vi "Assess Message Type.vi"(10 "Command Word":u16 format="%04x", 11 "Status Word":u16 format="%04x") -> (3 "Message Type":T1)   [LabVIEW 2016, in "BCI-1553 API.lvlib" / "Bus Monitor.lvclass"]
uses:
  Bus Monitor.lvclass
  TypeDefs/Bus Monitor Message Type.ctl
panel:
  out "test":u16 format="%016b"
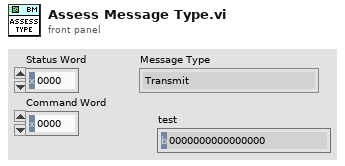
[diagram p1: front panel]
types:
  T1 = typedef "BCI-1553 API.lvlib/Bus Monitor.lvclass/Bus Monitor Message Type.ctl" = enum16{"Transmit", "Receive", "RT-RT Message", "Mode Code Transmit", "Mode Code Receive", "NULL"}
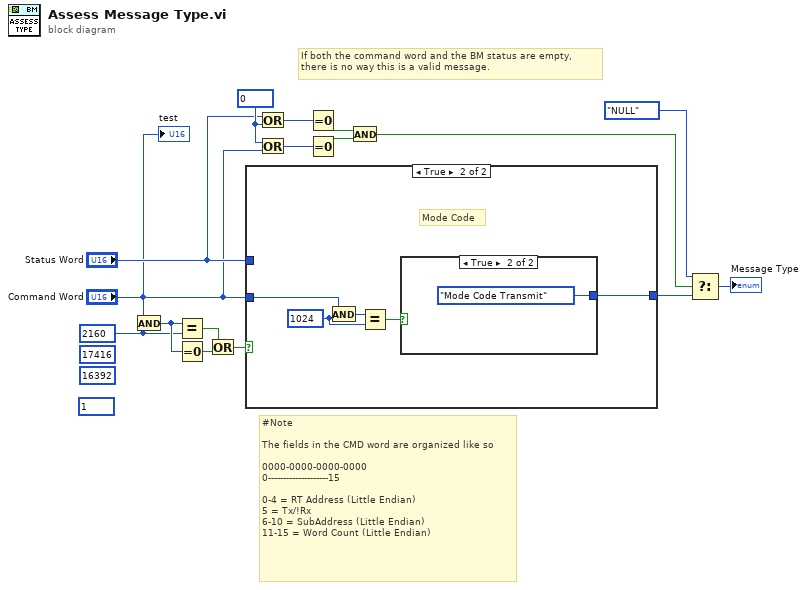
[diagram p0: block diagram]
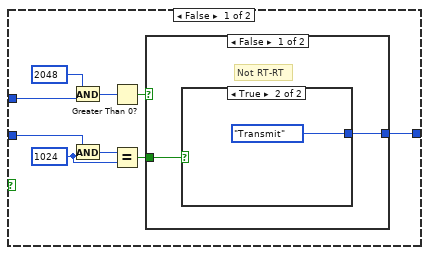
[diagram p2: hidden frame]
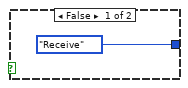
[diagram p3: hidden frame]
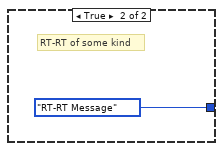
[diagram p4: hidden frame]
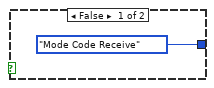
[diagram p5: hidden frame]
diagram:
  (unwired) u16 1 ("Numeric")
  (unwired) u16 16392 ("Numeric")
  (unwired) u16 17416 ("Numeric")
  w11 = u16 0 ("Numeric")
  w15 = u16 2160 ("Numeric")
  # "#Note\n\nThe fields in the CMD word are organized like so\n\n0000-0000-0000-0000\n0--------------------15\n\n0-4 = RT Address (Little Endian)\n5 = Tx/!Rx\n6-10 = SubAddress (Little Endian)\n11-15 = Word Count (Little Endian)"
  # "If both the command word and the BM status are empty,\nthere is no way this is a valid message."
  n1 = And(x="Command Word", y=w15) -> (x .and. y?=w16:u16)
  n2 = Equal?(x=w16, y=w15) -> (x = y?=w14:bool)
  n3 = Equal To 0?(x=w16) -> (x = 0?=w13:bool)
  n4 = Or(x=w14, y=w13) -> (x .or. y?=w12:bool)
  n5 = case shown="True" w12 {
    tunnel: "Status Word" -> [w25 _]
    tunnel: [w24 w31] -> w2
    tunnel: "Command Word" -> [w17 w33]
    frame False {
      w20 = u16 1024 ("Numeric")
      n6 = And(x=u16 2048 ("Numeric"), y=w25) -> (x .and. y?=w22:u16)
      n7 = And(x=w17, y=w20) -> (x .and. y?=w19:u16)
      n8 = Greater Than 0?(x=w22) -> (x > 0?=w21:bool)
      n9 = Equal?(x=w19, y=w20) -> (x = y?=w18:bool)
      n10 = case shown="False" w21 {
        tunnel: w18 -> [w27 _]
        tunnel: [w26 Bus_Monitor_Message_Type."RT-RT Message" ("Message Type")] -> w24
        frame False {
          # "Not RT-RT"
          n11 = case shown="True" w27 {
            tunnel: [Bus_Monitor_Message_Type."Receive" ("Message Type") Bus_Monitor_Message_Type."Transmit" ("Message Type")] -> w26
            frame False {
            }
            frame True {
            }
          }
        }
        frame True {
          # "RT-RT of some kind"
        }
      }
    }
    frame True {
      w35 = u16 1024 ("Numeric")
      # "Mode Code"
      n12 = And(x=w33, y=w35) -> (x .and. y?=w34:u16)
      n13 = Equal?(x=w34, y=w35) -> (x = y?=w32:bool)
      n14 = case shown="True" w32 {
        tunnel: [Bus_Monitor_Message_Type."Mode Code Receive" ("Message Type") Bus_Monitor_Message_Type."Mode Code Transmit" ("Message Type")] -> w31
        frame False {
        }
        frame True {
        }
      }
    }
  }
  n15 = Or(x="Status Word", y=w11) -> (x .or. y?=w8:u16)
  n16 = Or(x=w11, y="Command Word") -> (x .or. y?=w9:u16)
  n17 = Equal To 0?(x=w8) -> (x = 0?=w7:bool)
  n18 = Equal To 0?(x=w9) -> (x = 0?=w6:bool)
  n19 = And(x=w7, y=w6) -> (x .and. y?=w5:bool)
  n20 = Select(t=Bus_Monitor_Message_Type."NULL" ("Message Type"), s=w5, f=w2) -> (s? t:f=→"Message Type":T1)
  "test" <- "Command Word"
